vi "Process GPS Coordinates.vi"(11 "GPRMC-data":T1={"TimeStamp"=timestamp(0 s since 1904-01-01), "Validity"=FALSE, "Latitude"=0.0, "Latitude-Direction"=enum."North", "Longitude"=0.0, "Longitude-Direction"=enum."East", "Speed in knots"=0.0, "True course"=0.0, "Date Stamp"=timestamp(0 s since 1904-01-01), "Magnetic Variation (East/West)"=0.0, "GPS Latitude"=0.0, "GPS Longitude"=0.0} {"GPS Longitude" format="%.6f"; "GPS Latitude" format="%.6f"; "Magnetic Variation (East/West)" format="%.02f [deg]"; "Date Stamp" format="%<%x>T"; "True course" format="%.02f [deg]"; "Speed in knots" format="%.02f [kts]"; "Longitude" format="%0.4f [long]"; "Latitude" format="%.04f [lat]"; "TimeStamp" format="%<%.2X>T"}) -> (3 "GPRMC Data":T1={"TimeStamp"=timestamp(0 s since 1904-01-01), "Validity"=FALSE, "Latitude"=0.0, "Latitude-Direction"=enum."North", "Longitude"=0.0, "Longitude-Direction"=enum."East", "Speed in knots"=0.0, "True course"=0.0, "Date Stamp"=timestamp(0 s since 1904-01-01), "Magnetic Variation (East/West)"=0.0, "GPS Latitude"=0.0, "GPS Longitude"=0.0} {"GPS Longitude" format="%.6f"; "GPS Latitude" format="%.6f"; "Magnetic Variation (East/West)" format="%.02f [deg]"; "Date Stamp" format="%<%x>T"; "True course" format="%.02f [deg]"; "Speed in knots" format="%.02f [kts]"; "Longitude" format="%0.4f [long]"; "Latitude" format="%.04f [lat]"; "TimeStamp" format="%<%.2X>T"})   [LabVIEW 2015, in "GPS Instrument.lvlib" / "GPS Instrument.lvclass"]
uses:
  GPS Instrument.lvclass
  Libraries/3rd Party/NMEA_GPS/NMEA_GPRMC-data.ctl
  Libraries/3rd Party/NMEA_GPS/NMEA_LatitudeDirection.ctl
  Libraries/3rd Party/NMEA_GPS/NMEA_LongitudeDirection.ctl
  Libraries/3rd Party/NMEA_GPS/NMEA.lvlib
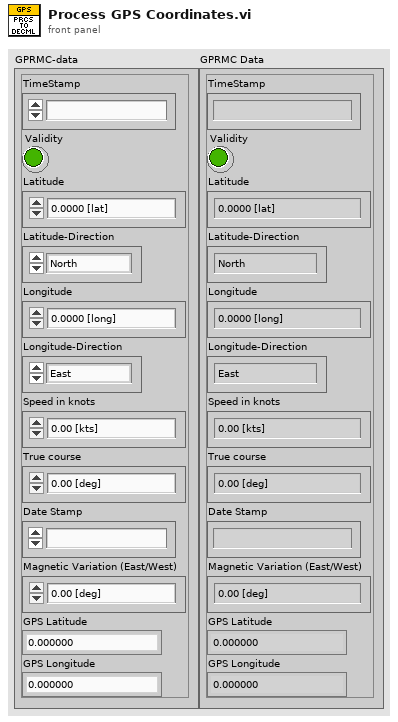
[diagram p1: front panel]
types:
  T1 = typedef "RDS Libraries.lvlib/NMEA.lvlib/NMEA_GPRMC-data.ctl" = cluster{"TimeStamp":timestamp, "Validity":bool, "Latitude":dbl, "Latitude-Direction":T2, "Longitude":dbl, "Longitude-Direction":T3, "Speed in knots":sgl, "True course":sgl, "Date Stamp":timestamp, "Magnetic Variation (East/West)":sgl, "GPS Latitude":dbl, "GPS Longitude":dbl}
  T2 = typedef "RDS Libraries.lvlib/NMEA.lvlib/NMEA_LatitudeDirection.ctl" = enum16{"", "North", "South"}
  T3 = typedef "RDS Libraries.lvlib/NMEA.lvlib/NMEA_LongitudeDirection.ctl" = enum16{"", "East", "West"}
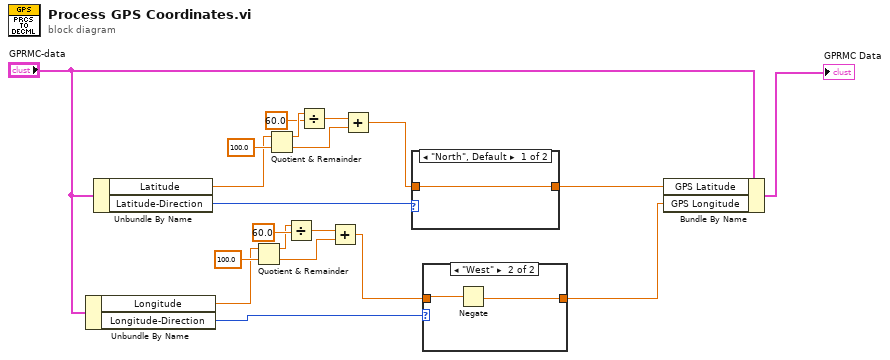
[diagram p0: block diagram]
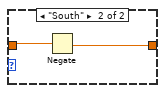
[diagram p3: hidden frame]
diagram:
  n1 = Unbundle By Name("GPRMC-data") -> ("Longitude"=w3:dbl, "Longitude-Direction"=w19:T3)
  n2 = Unbundle By Name("GPRMC-data") -> ("Latitude"=w11:dbl, "Latitude-Direction"=w20:T2)
  n3 = Quotient & Remainder(x=w3, y=100.0) -> (x-y*floor(x/y)=w6:dbl, floor(x/y)=w9:dbl)
  n4 = Quotient & Remainder(x=w11, y=100.0) -> (x-y*floor(x/y)=w15:dbl, floor(x/y)=w12:dbl)
  n5 = Divide(x=w6, y=60.0) -> (x/y=w8:dbl)
  n6 = Divide(x=w15, y=60.0) -> (x/y=w13:dbl)
  n7 = Add(x=w8, y=w9) -> (x+y=w4:dbl)
  n8 = Add(x=w13, y=w12) -> (x+y=w10:dbl)
  n9 = case shown="\"North\", Default" w20 {
    tunnel: w10 -> [w21 w23]
    tunnel: [w21 w22] -> w1
    frame "North", Default {
    }
    frame "South" {
      n10 = Negate(x=w23) -> (-x=w22:dbl)
    }
  }
  n11 = case shown="\"West\"" w19 {
    tunnel: w4 -> [w24 w26]
    tunnel: [w24 w25] -> w2
    frame "East", Default {
    }
    frame "West" {
      n12 = Negate(x=w26) -> (-x=w25:dbl)
    }
  }
  n13 = Bundle By Name(cluster="GPRMC-data", "GPS Latitude"=w1, "GPS Longitude"=w2) -> (→"GPRMC Data":T1)
